vi "Launch Module.vi"(8 "error in (no error)":errorcluster, 10 "Module Name":string="Module B") -> (0 "error out":errorcluster)   [LabVIEW 2018, in "Common.lvlib"]
uses:
  Common.lvlib
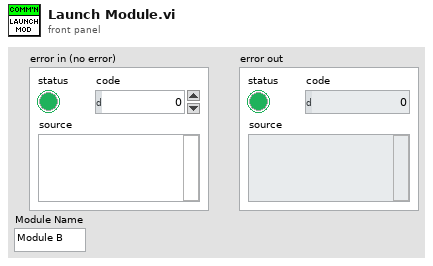
[diagram p1: front panel]
types:
  T1 = enum32{"Invalid", "Standard", "Closed", "Hidden", "Minimized", "Maximized"}
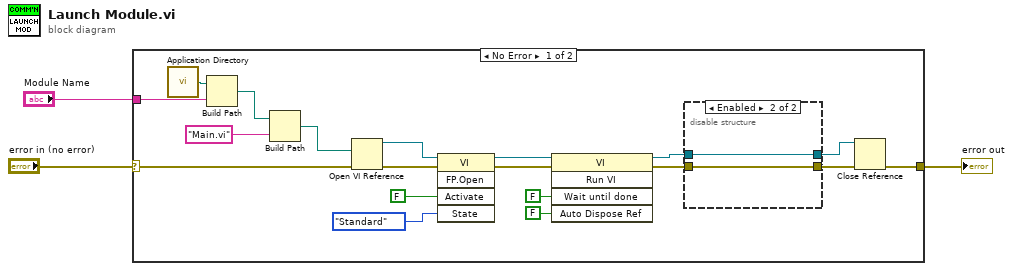
[diagram p0: block diagram]
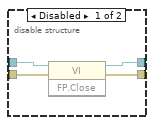
[diagram p2: hidden frame]
diagram:
  n1 = case shown="No Error" "error in (no error)" {
    selector: "error in (no error)" -> [w5 w29]
    tunnel: "Module Name" -> [w12 _]
    tunnel: [w4 w29] -> w1
    frame No Error {
      n2 = call <vilib>:"Application Directory.vi"() -> ("Application Directory"=w11:path)
      n3 = Build Path(base path=w11, name or relative path=w12) -> (appended path=w13:path)
      n4 = Build Path(base path=w13, name or relative path="Main.vi") -> (appended path=w15:path)
      n5 = Open VI Reference(vi path=w15, error in (no error)=w5) -> (vi reference=w16:refnum<vi>, error out=w9:errorcluster)  [unwired: 4 in]
      n6 = invoke class="VI" method="FP.Open"(reference=w16, error in=w9, "Activate"=FALSE ("Activate?"), "State"=T1."Standard") -> (reference out=w10:refnum<vi>, error out=w8:errorcluster)  [unwired: 1 in, 3 out]
      n7 = invoke class="VI" method="Run VI"(reference=w10, error in=w8, "Wait until done"=FALSE ("Wait Until Done"), "Auto Dispose Ref"=FALSE ("Auto Dispose Reference")) -> (reference out=w21:refnum<vi>, error out=w7:errorcluster)  [unwired: 1 in, 3 out]
      n8 = disable-structure shown="Enabled" {
        disable-tunnel: [w26 w28] -> w22
        disable-tunnel: w21 -> [w25 w28]
        disable-tunnel: w7 -> [w24 w27]
        disable-tunnel: [w23 w27] -> w6
        frame Disabled {
          n9 = invoke class="VI" method="FP.Close"(reference=w25, error in=w24) -> (reference out=w26:refnum<vi>, error out=w23:errorcluster)  [unwired: 1 in, 1 out]
        }
        frame Enabled {
        }
      }
      n10 = Close Reference(reference=w22, error in (no error)=w6) -> (error out=w4:errorcluster)
    }
    frame Error {
    }
  }
  "error out" <- w1
